vi "Datum_Image_Calibration.vi"(3 "Mode":T9=enum."Run VI", 5 "Traverse line In":T6={"Start X"=2159.9, "Start Y"=-208.7, "Start Z"=90.0, "End X"=nan, "End Y"=nan, "End Z"=nan, "No. of pts."=0, "Spacing"=enum."N/A", "Filename"=path "E:/Enflo_Data_Local/2016/EnFlo_Tunnel/Paul_Hayden/Calibrations/Cal_06-2016/Datum_Building.xls", "Tunnel Speed"=nan, "Averaging time (min)"=nan, "Extra Commands"="!Use_Axis_Correction  = X;Y", "Carrier_1 Q (l/min)"=nan, "Carrier_2 Q (l/min)"=nan, "Trace Gas Concentration (%)"=nan, "Specific Arguments"="Datum_Image_Calibration.vi;XYZ", "Comments"="", "Row No"=0, "Row Type Selector"=enum."Run VI Named:", "Completion time"="10:23  22-06-2016", "Row Duration (mins)"=0.08333333333333333, "No. of Valid pts."=0, "Meas Setup File"="Trav_Cam_Picture.xls"} {"Carrier_2 Q (l/min)" format="%#.2f"; "Row Duration (mins)" format="%#.1f"; "Row No" min=0; "Trace Gas Concentration (%)" min=0.0 format="%#_4f"; "Carrier_1 Q (l/min)" format="%#.4f"; "Tunnel Speed" format="%#.2f"; "Start X" format="%#.2f"; "Start Y" format="%#.2f"; "Start Z" format="%#.2f"; "End X" format="%#.2f"; "End Y" format="%#.2f"; "End Z" format="%#.2f"; "Averaging time (min)" min=0.0 format="%#.2f"}) -> (0 "Error Message":string, 1 "Status":T5, 2 "Traverse line Out":T6={"Start X"=2159.9, "Start Y"=-208.7, "Start Z"=90.0, "End X"=nan, "End Y"=nan, "End Z"=nan, "No. of pts."=0, "Spacing"=enum."N/A", "Filename"=path "E:/Enflo_Data_Local/2016/EnFlo_Tunnel/Paul_Hayden/Calibrations/Cal_06-2016/Datum_Building.xls", "Tunnel Speed"=nan, "Averaging time (min)"=nan, "Extra Commands"="!Use_Axis_Correction  = X;Y", "Carrier_1 Q (l/min)"=nan, "Carrier_2 Q (l/min)"=nan, "Trace Gas Concentration (%)"=nan, "Specific Arguments"="Datum_Image_Calibration.vi;XYZ", "Comments"="", "Row No"=0, "Row Type Selector"=enum."Run VI Named:", "Completion time"="10:23  22-06-2016", "Row Duration (mins)"=0.08333333333333333, "No. of Valid pts."=0, "Meas Setup File"="Trav_Cam_Picture.xls"} {"Carrier_2 Q (l/min)" format="%#.2f"; "Row Duration (mins)" format="%#.1f"; "Row No" min=0; "Trace Gas Concentration (%)" min=0.0 format="%#_4f"; "Carrier_1 Q (l/min)" format="%#.4f"; "Tunnel Speed" format="%#.2f"; "Start X" format="%#.2f"; "Start Y" format="%#.2f"; "Start Z" format="%#.2f"; "End X" format="%#.2f"; "End Y" format="%#.2f"; "End Z" format="%#.2f"; "Averaging time (min)" min=0.0 format="%#.2f"})   [LabVIEW 2018]
uses:
  Gen Trav/Traverse_cluster.ctl
  Gen Trav/Spacing.ctl
  Controls/Multi_run_mode.ctl
  Controls/User_Specific_mode.ctl
  Gen Trav/Multi_Run_Status.ctl
  Utilities/Image acquisition and processing/Feature detection/Typedefs/ROI bounds.ctl
  Utilities/Image acquisition and processing/Feature detection/Typedefs/Theta range.ctl
  Utilities/Image acquisition and processing/Feature detection/Typedefs/Txy range.ctl
  Utilities/Image acquisition and processing/Feature detection/Typedefs/Top level controls.ctl
  Gen Trav/Status_Cluster.ctl
  <vilib>/Analysis/baseanly.llb/Mean (DBL).vi
  Globals/Constants_global.vi
  Globals/Extra_Commands_Global.vi
  <vilib>/Analysis/NI_AALBase.lvlib
  <vilib>/Analysis/NI_AALPro.lvlib
panel:
  out "Camera":string
  out "intercept":dbl=-316.3339254329576
  out "slope":dbl=316.28786088822676
  out "Height calibration":cluster{dbl[], dbl[]}[](graph)
  out "Datum Type":string="XYZ"
  out "Setup file?":bool
  in  "Controls":T1={"Auto ROI (for rot.)"=FALSE, "Apply scaling"=FALSE, "Apply rotation"=FALSE, "Apply Tx"=TRUE, "Apply Ty"=TRUE, "Keep proc. img"=FALSE}
  in  "Txy range (pixels)":T2={"Tx max (pix)"=150, "Tx min (pix)"=-150, "Ty max (pix)"=150, "Ty min (pix)"=-150}
  in  "Theta range (deg)":T3={"theta max (deg)"=20.0, "theta min (deg)"=-20.0}
  in  "ROI to crop (pixels)":T4={"Xmax"=729, "Ymax"=464, "Xmin"=65, "Ymin"=76}
  out "Scale":dbl[](graph)
  out "Angle":dbl[](graph)
  out "Displacments":sgl[][](array[numeric])=[[-0.0, -0.0, -0.0], [-10.0, -0.0, -0.0], [10.0, -0.0, -0.0], [-0.0, -10.0, -0.0], [-0.0, 10.0, -0.0], [-0.0, -0.0, 10.0], [-0.0, -0.0, 5.0], [-0.0, -0.0, -5.0], [-0.0, -0.0, -10.0]]
  # "X           Y            Z"
  # "Start"
  # "End"
  # "X           Y            Z"
  # "Start"
  # "End"
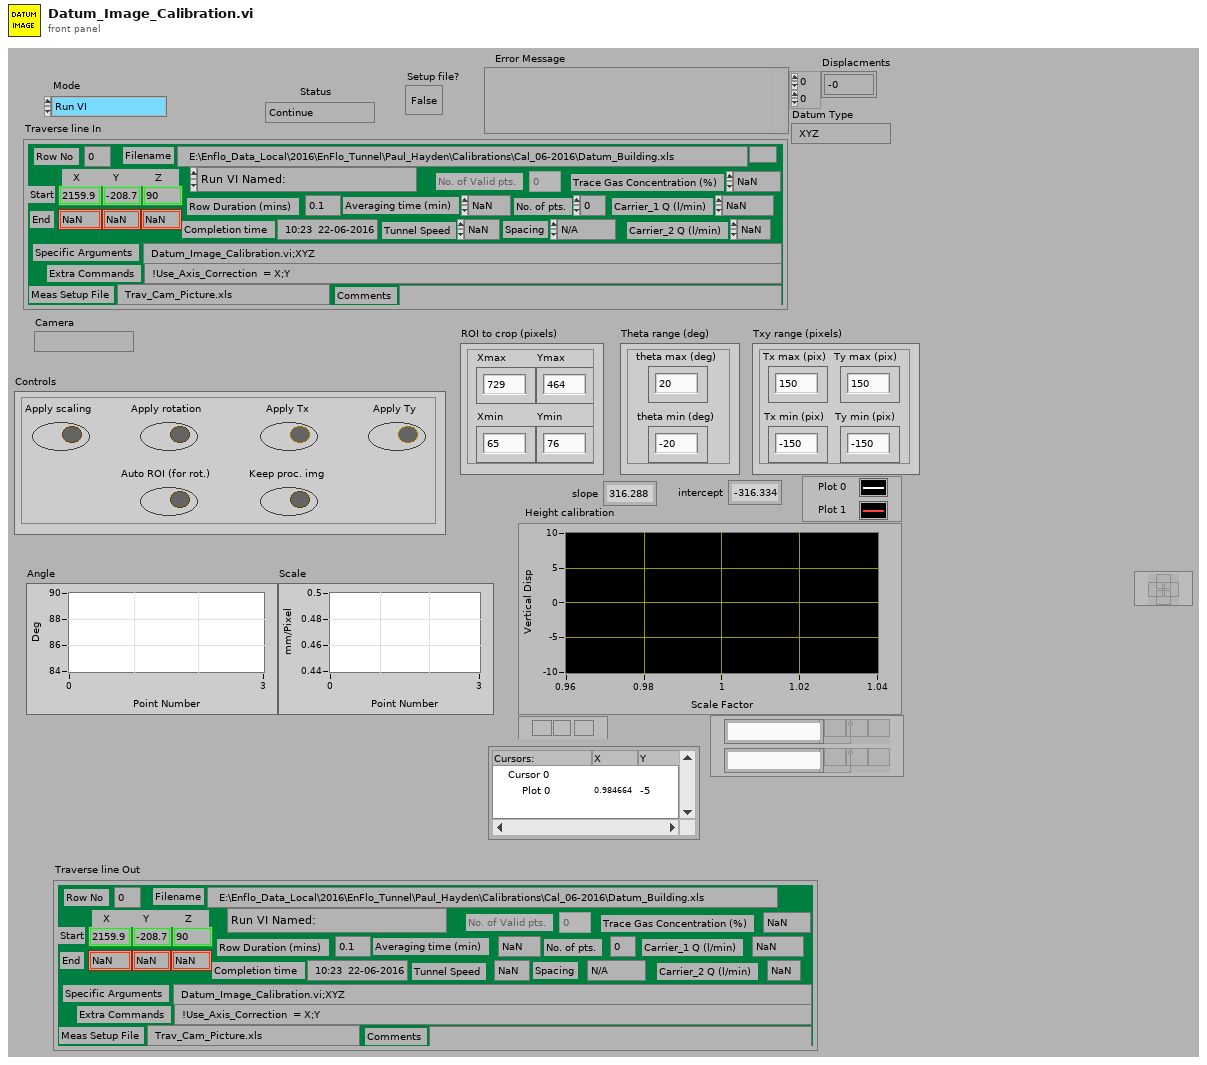
[diagram p1: front panel]
types:
  T1 = typedef "Top level controls.ctl" = cluster{"Auto ROI (for rot.)":bool, "Apply scaling":bool, "Apply rotation":bool, "Apply Tx":bool, "Apply Ty":bool, "Keep proc. img":bool}
  T2 = typedef "Txy range.ctl" = cluster{"Tx max (pix)":i32, "Tx min (pix)":i32, "Ty max (pix)":i32, "Ty min (pix)":i32}
  T3 = typedef "Theta range.ctl" = cluster{"theta max (deg)":dbl, "theta min (deg)":dbl}
  T4 = typedef "ROI bounds.ctl" = cluster{"Xmax":i32, "Ymax":i32, "Xmin":i32, "Ymin":i32}
  T5 = typedef "Multi_Run_Status.ctl" = enum16{"Continue", "Continue with Error", "Jump to Next Point", "Jump to Next Row", "Jump To Fall Back", "Terminate Run"}
  T6 = typedef "Traverse_cluster.ctl" = cluster{"Start X":sgl, "Start Y":sgl, "Start Z":sgl, "End X":sgl, "End Y":sgl, "End Z":sgl, "No. of pts.":i32, "Spacing":T7, "Filename":path, "Tunnel Speed":dbl, "Averaging time (min)":dbl, "Extra Commands":string, "Carrier_1 Q (l/min)":dbl, "Carrier_2 Q (l/min)":dbl, "Trace Gas Concentration (%)":dbl, "Specific Arguments":string, "Comments":string, "Row No":i32, "Row Type Selector":T8, "Completion time":string, "Row Duration (mins)":dbl, "No. of Valid pts.":i32, "Meas Setup File":string}
  T7 = typedef "Spacing.ctl" = enum16{"Linear", "Log", "Gauss", "Specified", "N/A"}
  T8 = typedef "Multi_run_mode.ctl" = enum16{"Move Traverse Only", "Set Tunnel Speed Only", "Set Source Only", "Set Measurement Conditions", "Single Measurement", "Vertical Profile", "Lateral Profile", "Longitudinal Profile", "Multi-Axis Profile", "Explore Volume", "Auto Calibrate", "Meas Fast FID Bkgnd", "Check Beam Power", "Scanning Valve Measurement", "Run VI Named:", "Set ADAM Ch", "Wait (minutes)", "Send Message", "Synchronize With:", "Fall Back to this Row", "Turn Off Row Repeating", "Traverse 3D Volume", "Blank Row", "Jump to Fall Back Row"}
  T9 = typedef "User_Specific_mode.ctl" = enum16{"Check VI only", "Run VI"}
  T10 = typedef "Status_Cluster.ctl" = cluster{"Status":T5, "Error Type":string, "Error Description":string}
  T11 = typedef "LVDateTimeRec.ctl" = cluster{"fractional second":dbl, "second":i32, "minute":i32, "hour":i32, "day of month":i32, "month":i32, "year":i32, "day of week":i32, "day of year":i32, "DST":i32}
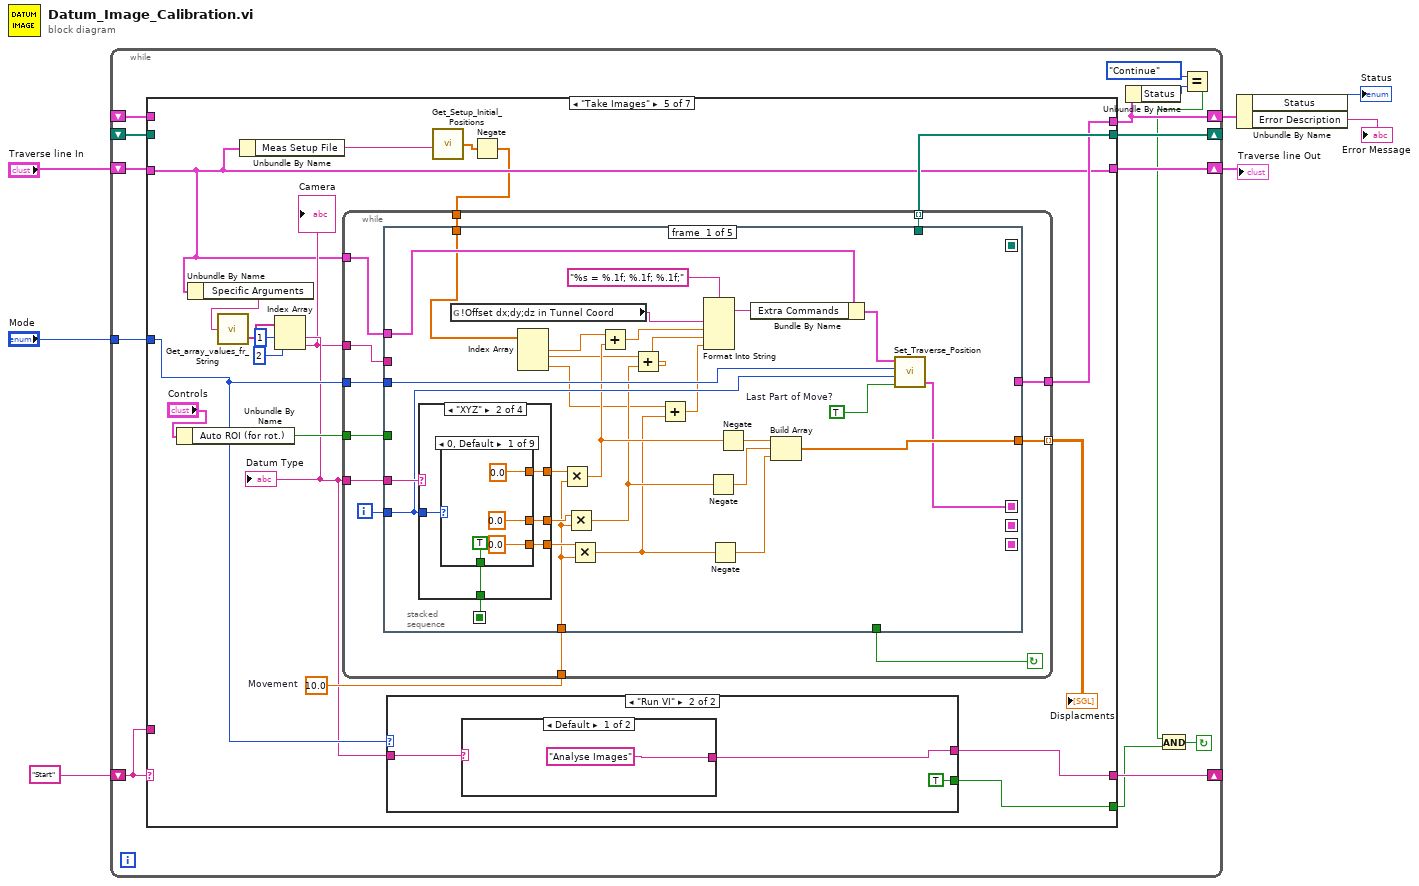
[diagram p0: block diagram]
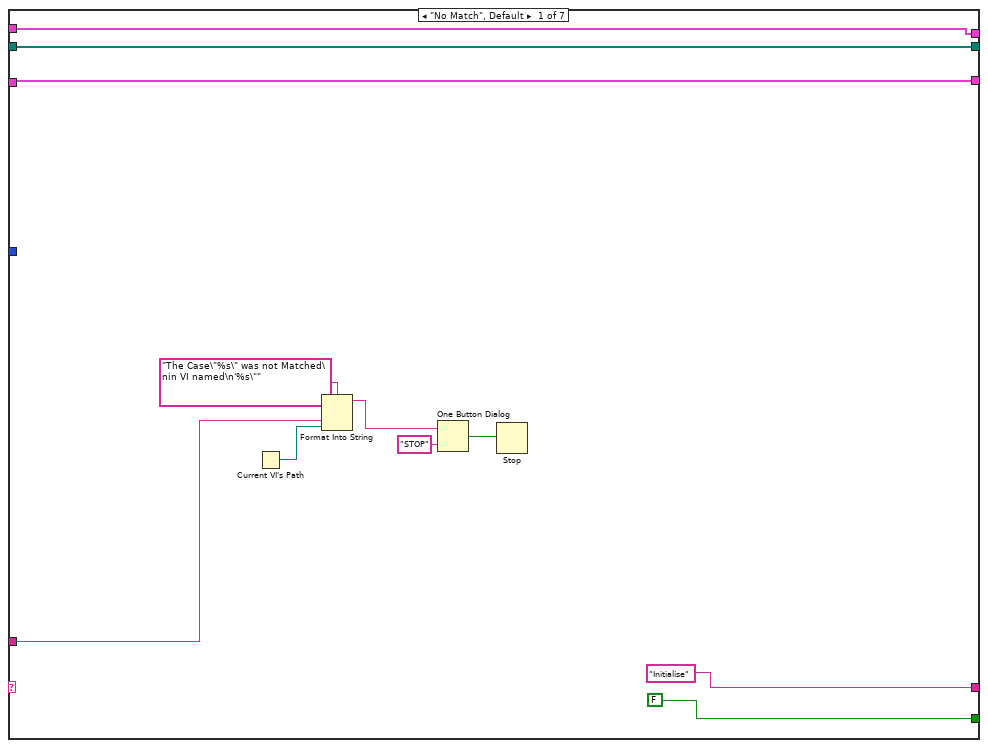
[diagram p2: hidden frame]
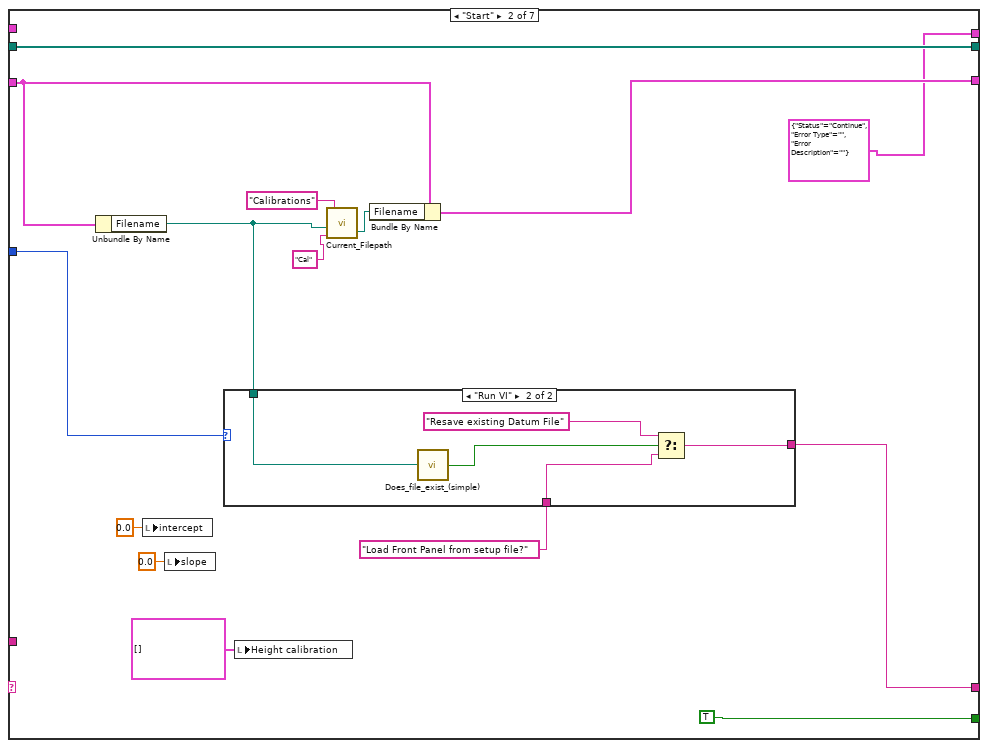
[diagram p3: hidden frame]
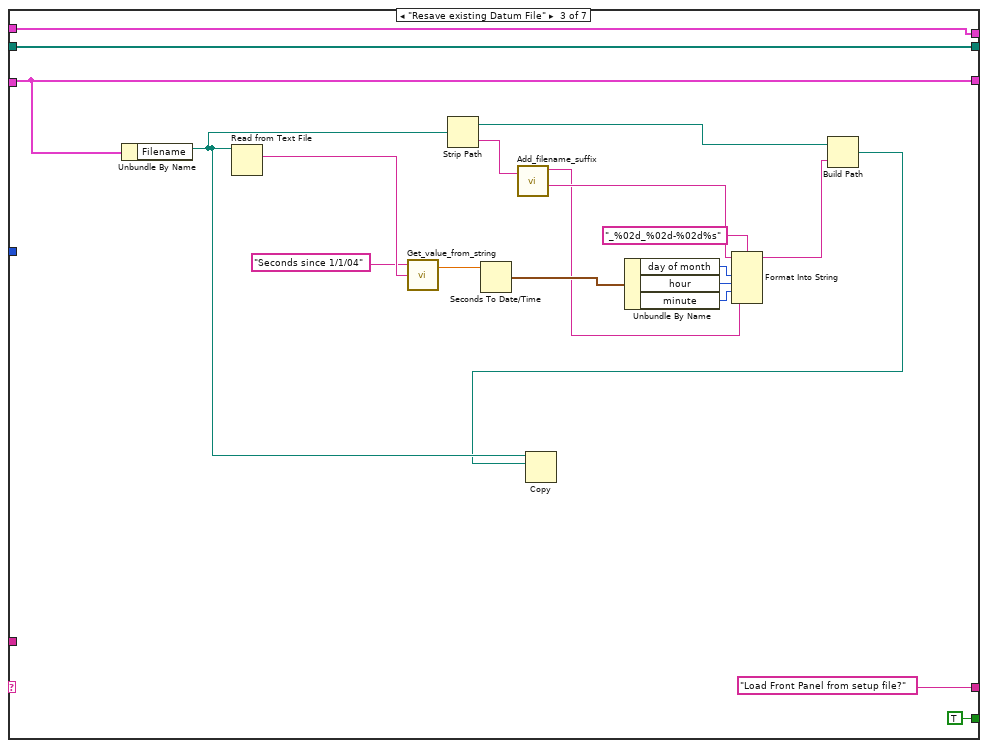
[diagram p5: hidden frame]
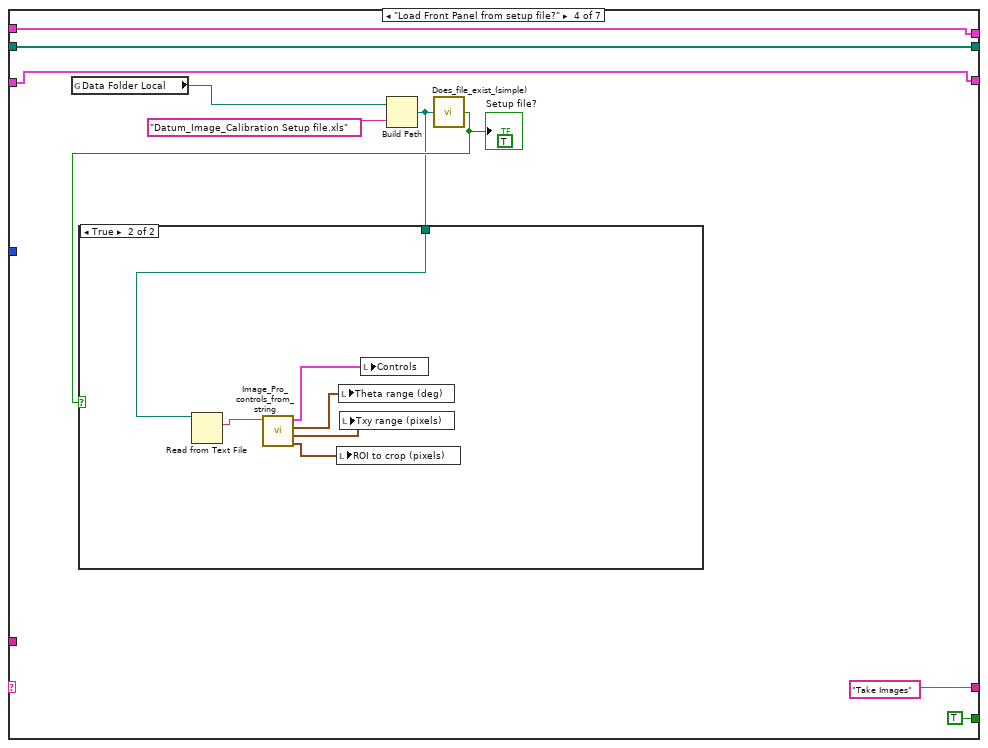
[diagram p6: hidden frame]
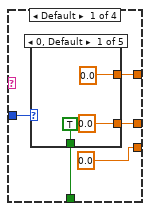
[diagram p8: hidden frame]
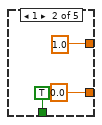
[diagram p9: hidden frame]
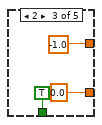
[diagram p10: hidden frame]
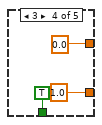
[diagram p11: hidden frame]
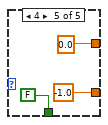
[diagram p12: hidden frame]
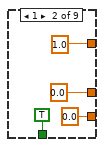
[diagram p13: hidden frame]
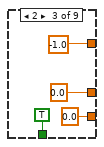
[diagram p14: hidden frame]
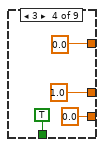
[diagram p15: hidden frame]
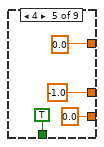
[diagram p16: hidden frame]
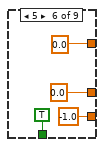
[diagram p17: hidden frame]
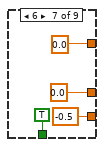
[diagram p18: hidden frame]
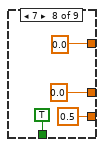
[diagram p19: hidden frame]
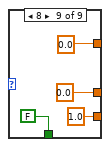
[diagram p20: hidden frame]
diagram:
  n1 = while {
    shift-left: "Start" -> [w20]
    shift-right: [w21] -> _
    tunnel: "Mode" -> [w19]
    shift-right: [w17] -> w4
    shift-left: "Traverse line In" -> [w18]
    shift-right: [w16] -> _
    shift-left: _ -> [w15]
    shift-right: [w14] -> w3
    shift-left: _ -> [w8]
    stop <- w10 continue-if-true
    n2 = case shown="\"Take Images\"" w20 {
      tunnel: [FALSE TRUE TRUE TRUE w104 TRUE FALSE] -> w11
      tunnel: ["Initialise" w36 "Load Front Panel from setup file?" "Take Images" w97 "Analyse Images" "Analyse Images"] -> w21
      tunnel: w20 -> [w27 _ _ _ _ _ _]
      tunnel: w19 -> [_ w39 _ _ w105 _ _]
      tunnel: w18 -> [w24 w44 w69 w75 w92 w329 w369]
      tunnel: [w24 w43 w69 w75 w92 w329 w369] -> w17
      tunnel: [w23 w42 w72 w76 w106 w335 w382] -> w16
      tunnel: w15 -> [w23 w42 w72 w76 _ w335 w382]
      tunnel: [w22 T10 {"Status"=enum."Continue", "Error Type"="", "Error Description"=""} ("Status Cluster Out") w73 w74 w99 w328 w356] -> w14
      tunnel: w8 -> [w22 _ w73 w74 _ w328 w356]
      frame "No Match", Default {
        n3 = Current VI's Path() -> (path=w26:path)
        n4 = Format Into String(format string="The Case\"%s\" was not Matched\nin VI named\n'%s\"" ("Format String"), w27, w26) -> (resulting string=w30:string)  [unwired: 2 in, 1 out]
        n5 = One Button Dialog(message=w30, button name ("OK")="STOP") -> (true=w28:bool)
        n6 = Stop(stop? (T)=w28) -> ()
      }
      frame "Start" {
        n7 = Unbundle By Name(w44) -> ("Filename"=w38:path)
        n8 = local write "intercept"(0.0 ("intercept")) -> ()
        n9 = local write "slope"(0.0 ("slope")) -> ()
        n10 = case shown="\"Run VI\"" w39 {
          tunnel: [w48 w51] -> w36
          tunnel: w38 -> [_ w50]
          tunnel: "Load Front Panel from setup file?" -> [w48 w49]
          frame "Check VI only" {
          }
          frame "Run VI" {
            n11 = call "Does_file_exist_(simple).vi"("Pathname"=w50) -> ("exists?"=w53:bool)
            n12 = Select(t="Resave existing Datum File", s=w53, f=w49) -> (s? t:f=w51:string)
          }
        }
        n13 = local write "Height calibration"(cluster{dbl[], dbl[]}[] [] ("Height calibration")) -> ()
        n14 = call "Current_Filepath.vi"("Short_Name"="Cal" ("Data Type"), "Filename in"=w38, "Data Type"="Calibrations") -> ("Filename Out"=w41:path)  [unwired: 1 in, 1 out]
        n15 = Bundle By Name(cluster=w44, "Filename"=w41) -> (w43:T6)
      }
      frame "Resave existing Datum File" {
        n16 = Unbundle By Name(w69) -> ("Filename"=w60:path)
        n17 = Read from Text File(file (use dialog)=w60) -> (text=w68:string)  [unwired: 3 in, 3 out]
        n18 = call "Get_value_from_string.vi"("Input string"=w68, "Variable name"="Seconds since 1/1/04") -> ("Value"=w66:dbl)  [unwired: 1 in, 1 out]
        n19 = Strip Path(path=w60) -> (stripped path=w59:path, name=w56:string)
        n20 = Seconds To Date/Time(time stamp (now)=w66) -> (date time rec=w65:T11)  [unwired: 1 in]
        n21 = call "Add_filename_suffix.vi"("Filename"=w56) -> ("Original Suffix"=w54:string, "Base name"=w55:string)  [unwired: 1 in, 2 out]
        n22 = Unbundle By Name(w65) -> ("day of month"=w64:i32, "hour"=w63:i32, "minute"=w62:i32)
        n23 = Format Into String(format string="_%02d_%02d-%02d%s", initial string=w55, w64, w63, w62, w54) -> (resulting string=w58:string)  [unwired: 1 in, 1 out]
        n24 = Build Path(base path=w59, name or relative path=w58) -> (appended path=w57:path)
        n25 = Copy(10:w57, 11:w60) -> ()  [unwired: 3 in, 3 out]
      }
      frame "Load Front Panel from setup file?" {
        (unwired) TRUE ("exists?")
        n26 = global read "Constants_global.vi" "Data Folder Local"() -> (w80:path)
        n27 = Build Path(base path=w80, name or relative path="Datum_Image_Calibration Setup file.xls") -> (appended path=w77:path)
        n28 = call "Does_file_exist_(simple).vi"("Pathname"=w77) -> ("exists?"=w78:bool)
        "Setup file?" <- w78
        n29 = case shown="True" w78 {
          tunnel: w77 -> [_ w88]
          frame False {
          }
          frame True {
            n30 = Read from Text File(file (use dialog)=w88) -> (text=w87:string)  [unwired: 3 in, 3 out]
            n31 = call "Image_Pro_controls_from_string.vi"("Setup String"=w87) -> ("ROI to crop (pixels)"=w83:T4, "Txy range (pixels)"=w84:T2, "Theta range (deg)"=w85:T3, "Controls"=w86:T1)  [unwired: 4 in, 3 out]
            n32 = local write "ROI to crop (pixels)"(w83) -> ()
            n33 = local write "Theta range (deg)"(w85) -> ()
            n34 = local write "Txy range (pixels)"(w84) -> ()
            n35 = local write "Controls"(w86) -> ()
          }
        }
      }
      frame "Take Images" {
        w107 = sgl 10.0  # Movement
        n36 = Unbundle By Name("Controls") -> ("Auto ROI (for rot.)"=w98:bool)
        n37 = Unbundle By Name(w92) -> ("Specific Arguments"=w102:string)
        n38 = call "Get_array_values_fr_String.vi"("String Value"=w102) -> ("String array"=w101:string[])  [unwired: 1 out]
        n39 = Unbundle By Name(w92) -> ("Meas Setup File"=w91:string)
        n40 = Index Array(array=w101, index #1=1 ("index"), index #2=2 ("index")) -> (element #1=w96:string, element #2=w93:string)
        "Datum Type" <- w96
        "Camera" <- w93
        n41 = case shown="\"Run VI\"" w105 {
          tunnel: [FALSE TRUE] -> w104
          tunnel: ["End" w304] -> w97
          tunnel: w96 -> [_ w305]
          frame "Check VI only" {
          }
          frame "Run VI" {
            n42 = case shown="Default" w305 {
              tunnel: ["Analyse Images" "Calculated Height Scaling"] -> w304
              frame Default {
              }
              frame "XYZ" {
              }
            }
          }
        }
        n43 = call "Get_Setup_Initial_Positions.vi"("Setup Filename"=w91) -> ("Initial Offsets"=w90:dbl[])
        n44 = Negate(x=w90) -> (-x=w89:dbl[])
        n45 = while {
          tunnel: w92 -> [w119]
          tunnel: w105 -> [w118]
          tunnel: w107 -> [w116]
          tunnel: [w115] -> w106 mode=indexing
          tunnel: [w114] -> w103 mode=indexing
          tunnel: w96 -> [w113]
          tunnel: [w111] -> w99
          tunnel: w98 -> [w110]
          tunnel: w93 -> [w109]
          tunnel: w89 -> [w108]
          i -> [w117]
          stop <- w112 continue-if-true
          n46 = stacked-sequence {
            seq-local: [_ _ w256 _ _] -> [_ _ _ w280 _]
            seq-local: [w139 _ _ _ _] -> [_ _ w254 w278 w301]
            seq-local: [_ _ w255 _ _] -> [_ _ _ _ w300]
            seq-local: [_ _ _ w279 _] -> [_ _ _ _ w298]
            seq-local: [w136 _ _ _ _] -> [_ _ _ _ w293]
            tunnel: w119 -> [w132 _ w258 _ _]
            tunnel: w118 -> [w148 w250 w257 w276 _]
            tunnel: w117 -> [w141 _ _ w283 _]
            tunnel: w116 -> [w137 _ _ _ _]
            tunnel: [_ _ w256 _ _] -> w115
            tunnel: [w145 _ _ _ _] -> w114
            tunnel: w113 -> [w142 _ _ _ _]
            tunnel: [_ _ _ _ w292] -> w112
            tunnel: [_ _ _ _ w295] -> w111
            tunnel: w110 -> [_ _ _ w274 _]
            tunnel: w109 -> [_ _ w253 _ _]
            tunnel: w108 -> [w129 _ _ _ _]
            frame #0 {
              w140 = TRUE  # Last Part of Move?
              n47 = case shown="\"XYZ\"" w142 {
                tunnel: w141 -> [w153 w173 w214 w234]
                tunnel: [w152 w172 w213 w233] -> w147
                tunnel: [w151 w171 w212 w232] -> w146
                tunnel: [sgl 0.0 ("Start Y") w170 sgl 0.0 ("Start Y") sgl 0.0 ("Start Y")] -> w138
                tunnel: [w149 w169 w210 w230] -> w136
                frame Default {
                  n48 = case shown="0, Default" w153 {
                    tunnel: [sgl 0.0 ("Start Y") sgl 1.0 ("Start Y") sgl -1.0 ("Start Y") sgl 0.0 ("Start Y") sgl 0.0 ("Start Y")] -> w152
                    tunnel: [sgl 0.0 ("Start Y") sgl 0.0 ("Start Y") sgl 0.0 ("Start Y") sgl 1.0 ("Start Y") sgl -1.0 ("Start Y")] -> w151
                    tunnel: [TRUE TRUE TRUE TRUE FALSE] -> w149
                    frame 0, Default {
                    }
                    frame 1 {
                    }
                    frame 2 {
                    }
                    frame 3 {
                    }
                    frame 4 {
                    }
                  }
                }
                frame "XYZ" {
                  n49 = case shown="0, Default" w173 {
                    tunnel: [sgl 0.0 ("Start Y") sgl 1.0 ("Start Y") sgl -1.0 ("Start Y") sgl 0.0 ("Start Y") sgl 0.0 ("Start Y") sgl 0.0 ("Start Y") sgl 0.0 ("Start Y") sgl 0.0 ("Start Y") sgl 0.0 ("Start Y")] -> w172
                    tunnel: [sgl 0.0 ("Start Y") sgl 0.0 ("Start Y") sgl 0.0 ("Start Y") sgl 1.0 ("Start Y") sgl -1.0 ("Start Y") sgl 0.0 ("Start Y") sgl 0.0 ("Start Y") sgl 0.0 ("Start Y") sgl 0.0 ("Start Y")] -> w171
                    tunnel: [sgl 0.0 ("Start Y") sgl 0.0 ("Start Y") sgl 0.0 ("Start Y") sgl 0.0 ("Start Y") sgl 0.0 ("Start Y") sgl -1.0 ("Start Y") sgl -0.5 ("Start Y") sgl 0.5 ("Start Y") sgl 1.0 ("Start Y")] -> w170
                    tunnel: [TRUE TRUE TRUE TRUE TRUE TRUE TRUE TRUE FALSE] -> w169
                    frame 0, Default {
                    }
                    frame 1 {
                    }
                    frame 2 {
                    }
                    frame 3 {
                    }
                    frame 4 {
                    }
                    frame 5 {
                    }
                    frame 6 {
                    }
                    frame 7 {
                    }
                    frame 8 {
                    }
                  }
                }
                frame "X Fixed" {
                  n50 = case shown="4" w214 {
                    tunnel: [sgl 0.0 ("Start Y") sgl 0.0 ("Start Y") sgl 0.0 ("Start Y") sgl 0.0 ("Start Y") sgl 0.0 ("Start Y")] -> w213
                    tunnel: [sgl 0.0 ("Start Y") sgl 0.5 ("Start Y") sgl 1.0 ("Start Y") sgl -0.5 ("Start Y") sgl -1.0 ("Start Y")] -> w212
                    tunnel: [TRUE TRUE TRUE TRUE FALSE] -> w210
                    frame 0, Default {
                    }
                    frame 1 {
                    }
                    frame 2 {
                    }
                    frame 3 {
                    }
                    frame 4 {
                    }
                  }
                }
                frame "Y Fixed" {
                  n51 = case shown="4" w234 {
                    tunnel: [sgl 0.0 ("Start Y") sgl 0.5 ("Start Y") sgl 1.0 ("Start Y") sgl -0.5 ("Start Y") sgl -1.0 ("Start Y")] -> w233
                    tunnel: [sgl 0.0 ("Start Y") sgl 0.0 ("Start Y") sgl 0.0 ("Start Y") sgl 0.0 ("Start Y") sgl 0.0 ("Start Y")] -> w232
                    tunnel: [TRUE TRUE TRUE TRUE FALSE] -> w230
                    frame 0, Default {
                    }
                    frame 1 {
                    }
                    frame 2 {
                    }
                    frame 3 {
                    }
                    frame 4 {
                    }
                  }
                }
              }
              n52 = global read "Extra_Commands_Global.vi" "!Offset dx;dy;dz in Tunnel Coord"() -> (w134:string)
              n53 = Index Array(array=w129) -> (element #1=w127:dbl, element #2=w125:dbl, element #3=w122:dbl)  [unwired: 3 in]
              n54 = Multiply(x=w147, y=w137) -> (x*y=w128:sgl)
              n55 = Multiply(x=w146, y=w137) -> (x*y=w124:sgl)
              n56 = Multiply(x=w138, y=w137) -> (x*y=w123:sgl)
              n57 = Add(x=w127, y=w128) -> (x+y=w126:dbl)
              n58 = Add(x=w125, y=w124) -> (x+y=w120:dbl)
              n59 = Add(x=w122, y=w123) -> (x+y=w121:dbl)
              n60 = Format Into String(format string="%s = %.1f; %.1f; %.1f;", w134, w126, w120, w121) -> (resulting string=w130:string)  [unwired: 2 in, 1 out]
              n61 = Negate(x=w124) -> (-x=w143:sgl)
              n62 = Negate(x=w123) -> (-x=w135:sgl)
              n63 = Negate(x=w128) -> (-x=w144:sgl)
              n64 = Bundle By Name(cluster=w132, "Extra Commands"=w130) -> (w131:T6)
              n65 = Build Array(w144, w143, w135) -> (w145:sgl[])
              n66 = call "Set_Traverse_Position.vi"("Last Part of Move?"=w140, "Currently on Point"=w141, "Simulate/Run"=w148, "Traverse line"=w131) -> ("Status Cluster"=w139:T10)  [unwired: 2 in]
            }
            frame #1 {
              n67 = case shown="\"Run VI\"" w250 {
                frame "Check VI only" {
                }
                frame "Run VI" {
                  n68 = call "Wait_Seconds_with_display.vi"("Message"="Waiting for Traverse to stop vibrating", "Seconds to wait"=10.0) -> ()  [unwired: 1 in, 1 out]
                }
              }
            }
            frame #2 {
              n69 = case shown="\"Run VI\"" w257 {
                tunnel: w258 -> [_ w271]
                tunnel: [path "" ("stripped path") w262] -> w256
                tunnel: [w259 w266] -> w255
                tunnel: w254 -> [w259 _]
                tunnel: w253 -> [_ w261]
                frame "Check VI only" {
                }
                frame "Run VI" {
                  n70 = Unbundle By Name(w271) -> ("Filename"=w269:path)
                  n71 = call "Get_Data_Base_file_code.vi"("Data Type"="Raw_Calibrations", "Results Filename"=w269, "Short_Name"="Raw_Cal" ("Data Type")) -> ("Raw Data File Name"=w268:path)  [unwired: 1 in, 3 out]
                  n72 = Strip Path(path=w268) -> (stripped path=w264:path, name=w270:string)
                  n73 = call "Add_filename_suffix.vi"("Filename"=w270) -> ("Base name"=w265:string)  [unwired: 1 in, 3 out]
                  n74 = call "Save_Single_Images_fr_iSpy.vi"("Image name"=w265, "Image directory path"=w264, "Camera"=w261) -> ("Error out"=w263:errorcluster, "Image Path"=w262:path)
                  n75 = call "Error_to_Status_Cluster.vi"("Error In"=w263, "Status"=Multi_Run_Status."Terminate Run") -> ("Status Cluster Out"=w266:T10)
                }
              }
            }
            frame #3 {
              n76 = Equal To 0?(x=w283) -> (x = 0?=w282:bool)
              n77 = Equal?(x=User_Specific_mode."Run VI" ("Mode"), y=w276) -> (x = y?=w275:bool)
              n78 = Compound Arithmetic op=AND(w275, invert w274, w282) -> (w281:bool)
              n79 = case shown="True" w281 {
                tunnel: w280 -> [_ w290]
                tunnel: [w284 w286] -> w279
                tunnel: w278 -> [w284 _]
                frame False {
                }
                frame True {
                  n80 = call "Draw ROI (user interactive).vi"("Dialog title message"="Please draw your region of interest rectangle", "Image file path"=w290) -> ("Error out"=w288:errorcluster, "ROI to crop (pixels)"=w289:T4)
                  n81 = case shown="No Error" w288 {
                    tunnel: w289 -> [w291 _]
                    frame No Error {
                      n82 = local write "ROI to crop (pixels)"(w291) -> ()
                    }
                    frame Error {
                    }
                  }
                  n83 = call "Error_to_Status_Cluster.vi"("Error In"=w288, "Status"=Multi_Run_Status."Terminate Run") -> ("Status Cluster Out"=w286:T10)
                }
              }
            }
            frame #4 {
              n84 = call "Merge_Status_Clusters.vi"("Status Cluster 2"=w300, "Status Cluster 1"=w301) -> ("Status Cluster Out"=w299:T10)
              n85 = call "Merge_Status_Clusters.vi"("Status Cluster 2"=w298, "Status Cluster 1"=w299) -> ("Status Cluster Out"=w295:T10)
              n86 = Unbundle By Name(w295) -> ("Status"=w296:T5)
              n87 = Equal?(x=Multi_Run_Status."Continue" ("Status"), y=w296) -> (x = y?=w294:bool)
              n88 = And(x=w294, y=w293) -> (x .and. y?=w292:bool)
            }
          }
        }
        "Displacments" <- w103
      }
      frame "Calculated Height Scaling" {
        w323 = TRUE ("Apply scaling")
        w324 = 5 ("index")
        n89 = local read "Controls"() -> (w322:T1)
        n90 = local read "Txy range (pixels)"() -> (w325:T2)
        n91 = local read "ROI to crop (pixels)"() -> (w326:T4)
        n92 = Bundle By Name(cluster=w322, "Apply scaling"=w323, "Apply rotation"=w323, "Apply Tx"=w323, "Apply Ty"=w323) -> (w321:T1)
        n93 = local read "Displacments"() -> (w334:sgl[][])
        n94 = local read "Theta range (deg)"() -> (w327:T3)
        n95 = Index Array(array=w335) -> (element=w330:path)  [unwired: 1 in]
        n96 = Array Subset(array=w335, index=w324) -> (w332:path[])  [unwired: 1 in]
        n97 = Array Subset(array=w334, index (row)=w324) -> (w333:sgl[][])  [unwired: 3 in]
        n98 = for {
          tunnel: w333 -> [w350] mode=indexing
          tunnel: w330 -> [w349]
          tunnel: w332 -> [w348] mode=indexing
          tunnel: w326 -> [w347]
          tunnel: w325 -> [w344]
          tunnel: w327 -> [w343]
          tunnel: w321 -> [w342]
          tunnel: [w340] -> w320 mode=indexing
          tunnel: [w339] -> w317 mode=indexing
          w337 = 200.0  # R_min
          w338 = 0  # Pre-scale iters
          n99 = call "Image roto-translation top level.vi"("ROI to crop (pixels)"=w347, "Theta range (deg)"=w343, "Txy range (pixels)"=w344, "Controls"=w342, "Test image file path"=w348, "R_min"=w337, "Reference image file path"=w349, "Pre-scale iters"=w338) -> ("Scale factor"=w340:dbl, "Error Out"=w345:errorcluster)  [unwired: 4 in, 6 out]
          n100 = Index Array(array=w350, index=2) -> (element=w339:sgl)
          n101 = call "EnFlo_Error_Handler.vi"("error in (no error)"=w345, "Dialog Box (T)"=FALSE) -> ()  [unwired: 1 in, 3 out]
        }
        n102 = Build Array (concatenate)(1.0 ("Scale factor"), w320) -> (w312:dbl[])
        n103 = Build Array (concatenate)(0.0 ("Scale factor"), w317) -> (w314:dbl[])
        n104 = Bundle(w312, w314) -> (w316:cluster{dbl[], dbl[]})  [unwired: 1 in]
        n105 = call <vilib>:"Linear Fit.vi"("Y"=w314, "X"=w312) -> ("Best Linear Fit"=w313:dbl[], "slope"=→"slope":dbl, "intercept"=→"intercept":dbl)  [unwired: 9 in, 2 out]
        n106 = Bundle(w312, "Best Linear Fit"=w313) -> (w311:cluster{dbl[], "Best Linear Fit":dbl[]})  [unwired: 1 in]
        n107 = Build Array(w316, w311) -> (→"Height calibration":cluster{dbl[], "Best Linear Fit":dbl[]}[])
      }
      frame "Analyse Images" {
        w357 = dbl[] []
        (unwired) T3 {"theta max (deg)"=180.0, "theta min (deg)"=-180.0} ("Theta range (deg)")
        w353 = 1 ("index")
        n108 = local read "Controls"() -> (w354:T1)
        n109 = local read "Displacments"() -> (w381:sgl[][])
        n110 = Index Array(array=w382) -> (element=w377:path)  [unwired: 1 in]
        n111 = Array Subset(array=w382, index=w353) -> (w379:path[])  [unwired: 1 in]
        n112 = Array Subset(array=w381, index (row)=w353) -> (w380:sgl[][])  [unwired: 3 in]
        n113 = Unbundle By Name(w369) -> ("Filename"=w376:path)
        n114 = for {
          N: 4 -> [_]
          tunnel: w380 -> [w451] mode=indexing
          tunnel: w377 -> [w448]
          tunnel: w379 -> [w447] mode=indexing
          tunnel: "ROI to crop (pixels)" -> [w446]
          tunnel: "Txy range (pixels)" -> [w443]
          tunnel: "Theta range (deg)" -> [w442]
          tunnel: w354 -> [w440]
          shift-right: [w435] -> w361
          shift-left: w357 -> [w436]
          shift-right: [w434] -> w362
          shift-left: w357 -> [w437]
          w432 = 115.0  # R_min
          w433 = 2  # Pre-scale iters
          # "Mirror axis to allow rotation"
          n115 = call "Image roto-translation top level.vi"("ROI to crop (pixels)"=w446, "Theta range (deg)"=w442, "Txy range (pixels)"=w443, "Controls"=w440, "Test image file path"=w447, "R_min"=w432, "Reference image file path"=w448, "Pre-scale iters"=w433) -> ("Tx (pixels)"=w441:dbl, "Ty (pixels)"=w431:dbl, "Error Out"=w444:errorcluster)  [unwired: 4 in, 5 out]
          n116 = Index Array(array=w451) -> (element #1=w450:sgl, element #2=w449:sgl)  [unwired: 2 in]
          n117 = Negate(x=w431) -> (-x=w430:dbl)
          n118 = call "EnFlo_Error_Handler.vi"("error in (no error)"=w444, "Dialog Box (T)"=FALSE) -> ()  [unwired: 1 in, 3 out]
          n119 = call "Get camera angle and scale factor from trav moves.vi"("dy (pix)"=w430, "dx (pix)"=w441, "dy (mm)"=w449, "dx (mm)"=w450) -> ("scale factor (mm / pixel)"=w438:dbl, "camera angle, ccw+ rel. to trav. (deg)"=w439:dbl)
          n120 = Build Array (concatenate)(w436, w439) -> (w435:dbl[])
          "Angle" <- w435
          n121 = Build Array (concatenate)(w437, w438) -> (w434:dbl[])
          "Scale" <- w434
        }
        n122 = Array Max & Min(array=w362) -> (max value=w365:dbl, min value=w363:dbl)  [unwired: 2 out]
        n123 = call-poly <vilib>:"Mean.vi"("X"=w361) -> ("mean"=w375:dbl)  [unwired: 1 out]
        n124 = call-poly <vilib>:"Mean.vi"("X"=w362) -> ("mean"=w364:dbl)  [unwired: 1 out]
        n125 = Subtract(x=w364, y=w363) -> (x-y=w359:dbl)
        n126 = Subtract(x=w365, y=w364) -> (x-y=w360:dbl)
        n127 = Max & Min(x=w360, y=w359) -> (max(x,y)=w358:dbl)  [unwired: 1 out]
        n128 = Divide(x=w358, y=w364) -> (x/y=w368:dbl)
        n129 = Multiply(x=100.0, y=w368) -> (x*y=w351:dbl)
        n130 = stacked-sequence {
          seq-local: [w393 _ _ _] -> [_ _ _ w428]
          seq-local: [_ _ w412 _] -> [_ _ _ w427]
          seq-local: [_ w403 _ _] -> [_ _ w411 _]
          tunnel: w377 -> [w399 _ _ _]
          tunnel: w375 -> [w394 _ _ _]
          tunnel: w364 -> [w392 _ _ _]
          tunnel: "ROI to crop (pixels)" -> [_ _ w415 _]
          tunnel: [_ _ _ w429] -> w373
          tunnel: "Theta range (deg)" -> [_ _ w414 _]
          tunnel: "Txy range (pixels)" -> [_ _ w413 _]
          tunnel: w354 -> [_ w405 _ _]
          tunnel: w351 -> [_ _ _ w418]
          frame #0 {
            n131 = call "Path_2_String.vi"("Real Path"=w399) -> ("Path String"=w400:string)
            n132 = call "Value_to_string.vi"("Value"=w394, "Label for value"="Camera Angle") -> ("Output string"=w396:string)  [unwired: 1 in]
            n133 = call "Date_and_Time_to_string.vi"() -> ("Date and time (spreadsheet)"=w395:string)
            n134 = call "Value_to_string.vi"("Value"=w392, "Label for value"="scale factor (mm / pixel)") -> ("Output string"=w397:string)  [unwired: 1 in]
            n135 = call "Characters_to_string.vi"("Characters to write"=w400, "Label for characters"="Datum Image Filename") -> ("Output string"=w391:string)
            n136 = Concatenate Strings(w395, w396, w397, w391) -> (w393:string)
          }
          frame #1 {
            n137 = local read "Datum Type"() -> (w404:string)
            n138 = case shown="\"XYZ\"" w404 {
              tunnel: w405 -> [w406 w409]
              tunnel: [w406 w408] -> w403
              frame Default {
              }
              frame "XYZ" {
                w407 = TRUE ("Apply scaling")
                n139 = Bundle By Name(cluster=w409, "Apply scaling"=w407, "Apply rotation"=w407, "Apply Tx"=w407, "Apply Ty"=w407) -> (w408:T1)
              }
            }
          }
          frame #2 {
            n140 = local read "Camera"() -> (w410:string)
            n141 = call "Image_Pro_controls_to_string.vi"("Camera"=w410, "ROI to crop (pixels)"=w415, "Txy range (pixels)"=w413, "Theta range (deg)"=w414, "Controls"=w411) -> ("Setup String"=w412:string)  [unwired: 6 in]
          }
          frame #3 {
            w422 = "3" ("precision")
            n142 = local read "intercept"() -> (w420:dbl)
            n143 = local read "slope"() -> (w421:dbl)
            n144 = call "Value_to_string.vi"("precision"=w422, "Value"=w420, "Label for value"="Object_Height_Offset") -> ("Output string"=w423:string)
            n145 = call "Value_to_string.vi"("precision"=w422, "Value"=w421, "Label for value"="Object_Height_Gradient") -> ("Output string"=w424:string)
            n146 = call "Value_to_string.vi"("precision"="1", "Value"=w418, "Label for value"="% Variation in scale factor") -> ("Output string"=w417:string)
            n147 = Concatenate Strings(w428, w427, w424, w423, w417) -> (w429:string)
          }
        }
        n148 = Write to Text File(file (use dialog)=w376, text=w373) -> ()  [unwired: 2 in, 3 out]
        n149 = Greater?(x=w351, y=3.0) -> (0:w370:bool)
        n150 = case shown="True" w370 {
          tunnel: w351 -> [_ w390]
          tunnel: "\nThe variation in scale factor of the datum image is %.1f %%." ("format string") -> [_ w389]
          frame False {
          }
          frame True {
            n151 = Format Into String(format string=w389, w390) -> (resulting string=w386:string)  [unwired: 2 in, 1 out]
            n152 = Bundle By Name(cluster=errorcluster {"status"=FALSE, "code"=0, "source"=""} ("error in (no error)"), "status"=TRUE, "source"=w386) -> (w384:errorcluster)
            n153 = call "EnFlo_Error_Handler.vi"("error in (no error)"=w384, "Dialog Box (T)"=FALSE) -> ()  [unwired: 1 in, 3 out]
          }
        }
      }
    }
    n154 = Unbundle By Name(w14) -> ("Status"=w13:T5)
    n155 = Equal?(x=Multi_Run_Status."Continue" ("Status"), y=w13) -> (x = y?=w9:bool)
    n156 = And(x=w9, y=w11) -> (x .and. y?=w10:bool)
  }
  "Traverse line Out" <- w4
  n157 = Unbundle By Name(w3) -> ("Status"=→"Status":T5, "Error Description"=→"Error Message":string)
